vi "PADMINI_AUTO_CYCLE STATE 60.vi"(7 "Enum":enum16{"Read", "Write"}(ring), 8 "error in (no error)":errorcluster, 11 "Input":bool[](array[boolean])) -> (0 "error out":errorcluster, 3 "Input 2":bool[](array[boolean]))   [LabVIEW 2017]
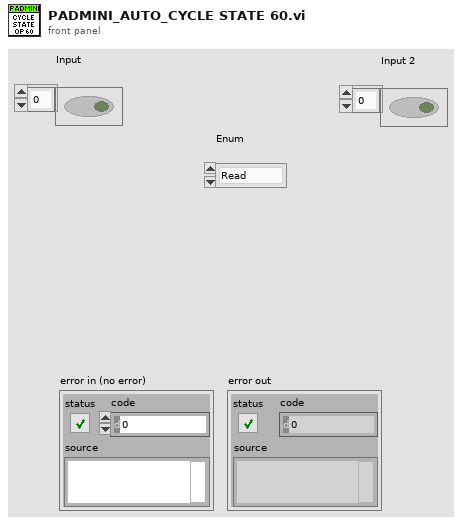
[diagram p1: front panel]
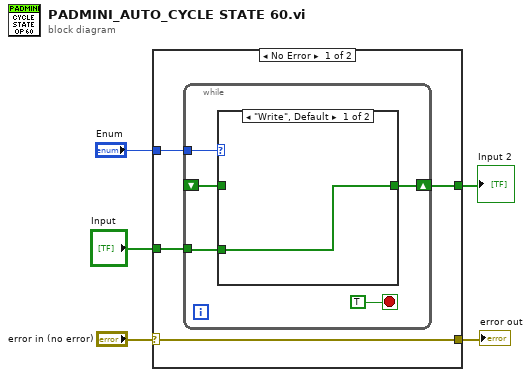
[diagram p0: block diagram]
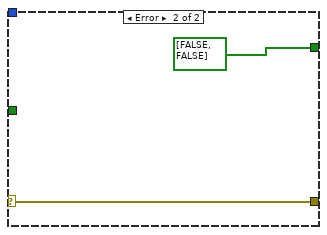
[diagram p3: hidden frame]
diagram:
  n1 = case shown="No Error" "error in (no error)" {
    selector: "error in (no error)" -> [w6 w17]
    tunnel: "Enum" -> [w9 _]
    tunnel: "Input" -> [w8 _]
    tunnel: [w7 bool[] [FALSE, FALSE]] -> w1
    tunnel: [w6 w17] -> w3
    frame No Error {
      n2 = while {
        tunnel: w9 -> [w14]
        shift-right: [w12] -> w7
        shift-left: _ -> [w11]
        tunnel: w8 -> [w13]
        stop <- TRUE stop-if-true
        n3 = case shown="\"Write\", Default" w14 {
          tunnel: [w15 w16] -> w12
          tunnel: w13 -> [w15 _]
          tunnel: w11 -> [_ w16]
          frame "Write", Default {
          }
          frame "Read" {
          }
        }
      }
    }
    frame Error {
    }
  }
  "Input 2" <- w1
  "error out" <- w3
